vi "AD7747_Hex to Cap Converter.vi"(8 "?":errorcluster, 11 "HEX":string) -> (0 "?":errorcluster, 2 "DEC":dbl, 3 "CAP (pF)":dbl)   [LabVIEW 2017]
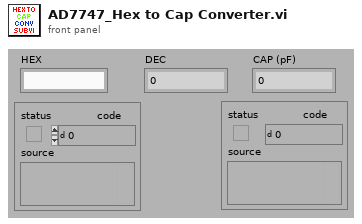
[diagram p1: front panel]
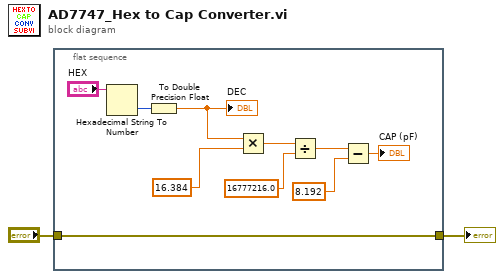
[diagram p0: block diagram]
diagram:
  n1 = flat-sequence {
    tunnel: "?" -> [w5]
    tunnel: [w5] -> w1
    frame #0 {
      n2 = Hexadecimal String To Number(string="HEX") -> (number=w4:u32)  [unwired: 2 in, 1 out]
      n3 = To Double Precision Float(number=w4) -> (double precision float=w3:dbl)
      "DEC" <- w3
      n4 = Multiply(x=w3, y=16.384) -> (x*y=w11:dbl)
      n5 = Divide(x=w11, y=16777216.0) -> (x/y=w9:dbl)
      n6 = Subtract(x=w9, y=8.192) -> (x-y=→"CAP (pF)":dbl)
    }
  }
  "?" <- w1
